vi "信号发生器.vi"() -> ()   [LabVIEW 2020]
uses:
  <vilib>/measure/NI_MABase.lvlib
panel:
  in  "stop (F)":bool
  in  "sampling info":cluster{"Fs":dbl, "#s":dbl}={"Fs"=10000.0, "#s"=1000.0} {"Fs" format="%.2p"}
  in  "amplitude":dbl=1.0 format="%0.2p"
  in  "frequency":dbl=10.0 format="%0.2p"
  in  "signal type":T1(ring)
  out "Waveform Graph":waveform(dbl)(graph)
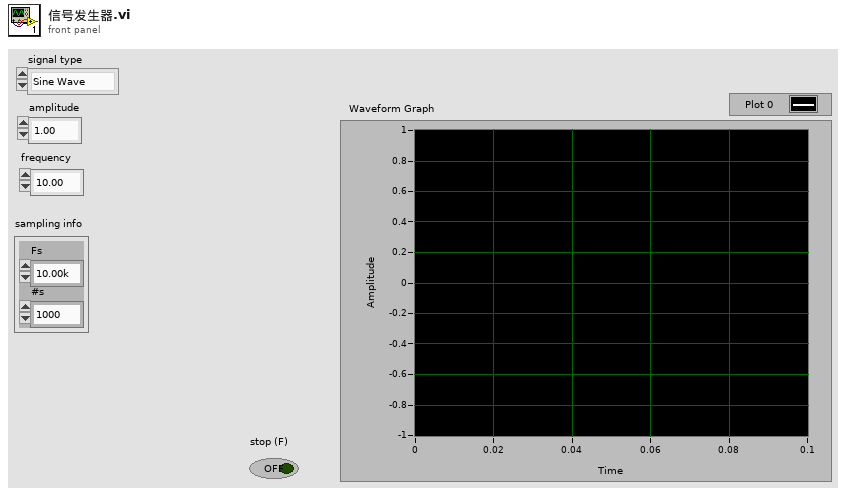
[diagram p1: front panel]
types:
  T1 = enum16{"Sine Wave", "Triangle Wave", "Square Wave", "Sawtooth Wave"}
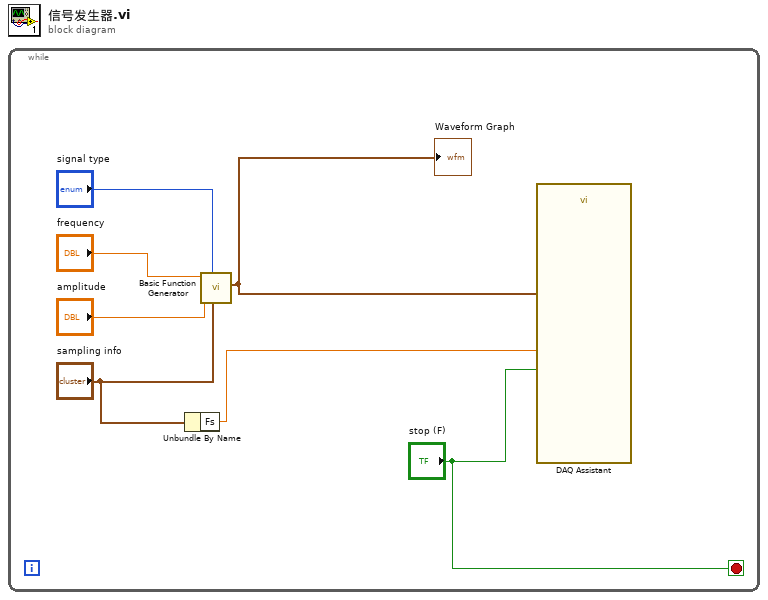
[diagram p0: block diagram]
diagram:
  n1 = while {
    stop <- "stop (F)" stop-if-true
    n2 = Unbundle By Name "Unbundle By Name"("sampling info") -> ("Fs"=w2:dbl)
    n3 = call <vilib>:"Basic Function Generator.vi"("sampling info"="sampling info", "signal type"="signal type", "amplitude"="amplitude", "frequency"="frequency") -> ("signal out"=w4:waveform(dbl))  [unwired: 5 in, 2 out]
    "Waveform Graph" <- w4
    n4 = call "DAQ Assistant"("data"=w4, "rate"=w2, "stop (F)"="stop (F)") -> ()  [unwired: 14 in, 3 out]
  }
